vi "Read.vi"(7 "error in":errorcluster, 10 "VISA resource name":refnum<visa-resource-name>) -> (0 "error out":errorcluster, 2 "String":string)   [LabVIEW 2017]
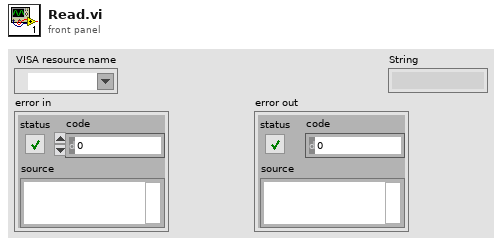
[diagram p1: front panel]
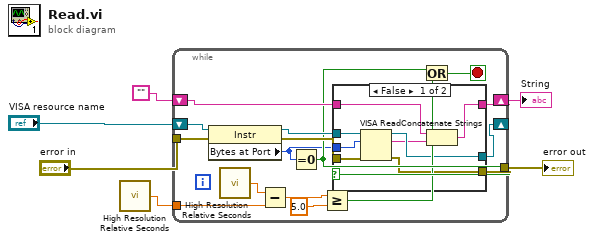
[diagram p0: block diagram]
diagram:
  n1 = call <vilib>:"High Resolution Relative Seconds.vi"() -> ("relative seconds"=w5:dbl)
  n2 = while {
    shift-right: [w21] -> _
    shift-left: "VISA resource name" -> [w20]
    tunnel: [w22] -> w1
    tunnel: "error in" -> [w18]
    shift-right: [w16] -> w2
    shift-left: "" -> [w17]
    tunnel: w5 -> [w10]
    stop <- w12 stop-if-true
    n3 = property class="Instr"(reference=w20, error in=w18) -> (reference out=w19:refnum<visa-resource-name>, error out=w15:errorcluster, "Bytes at Port"=w13:u32)
    n4 = call <vilib>:"High Resolution Relative Seconds.vi"() -> ("relative seconds"=w11:dbl)
    n5 = Subtract(x=w11, y=w10) -> (x-y=w9:dbl)
    n6 = Equal To 0?(x=w13) -> (x = 0?=w14:bool)
    n7 = Greater Or Equal?(x=w9, y=5.0 ("x")) -> (x >= y?=w7:bool)
    n8 = case shown="False" w14 {
      tunnel: [w30 w31] -> w22
      tunnel: [w29 w32] -> w21
      tunnel: w19 -> [w28 w32]
      tunnel: w17 -> [w26 w33]
      tunnel: [w25 w33] -> w16
      tunnel: w15 -> [w24 w31]
      tunnel: w13 -> [w23 _]
      frame False {
        n9 = VISA Read(VISA resource name=w28, byte count=w23, error in (no error)=w24) -> (VISA resource name out=w29:refnum<visa-resource-name>, read buffer=w27:string, error out=w30:errorcluster)  [unwired: 1 out]
        n10 = Concatenate Strings(w26, w27) -> (w25:string)
      }
      frame True {
      }
    }
    n11 = Or(x=w14, y=w7) -> (x .or. y?=w12:bool)
  }
  "String" <- w2
  "error out" <- w1
